vi "Errorbar0007.vi"   [LabVIEW 2013]
uses:
  <vilib>/Heliosphere Research LLC/Advanced Plotting Toolkit/api_plotting/ErrorbarProperties.ctl
  <vilib>/Heliosphere Research LLC/Advanced Plotting Toolkit/typedefs/PlotColor.ctl
  <vilib>/Heliosphere Research LLC/Advanced Plotting Toolkit/properties/Display.ctl
  <vilib>/Heliosphere Research LLC/Advanced Plotting Toolkit/api_core/NewPlotScales.ctl
  <vilib>/Heliosphere Research LLC/Advanced Plotting Toolkit/Advanced Plotting Toolkit.lvlib
types:
  T1 = typedef "Advanced Plotting Toolkit.lvlib/NewPlotScales.ctl" = enum16{"Default", "Linear", "Log", "Symlog"}
  T2 = typedef "Advanced Plotting Toolkit.lvlib/ErrorbarProperties.ctl" = cluster{"Color":T3, "Line Width":dbl, "Cap Size":dbl, "Display":T4}
  T3 = typedef "Advanced Plotting Toolkit.lvlib/PlotColor.ctl" = u32
  T4 = typedef "Advanced Plotting Toolkit.lvlib/Display.ctl" = cluster{"Alpha":dbl, "Z Order":dbl}
  T5 = typedef "Advanced Plotting Toolkit.lvlib/PlotID.ctl" = i32
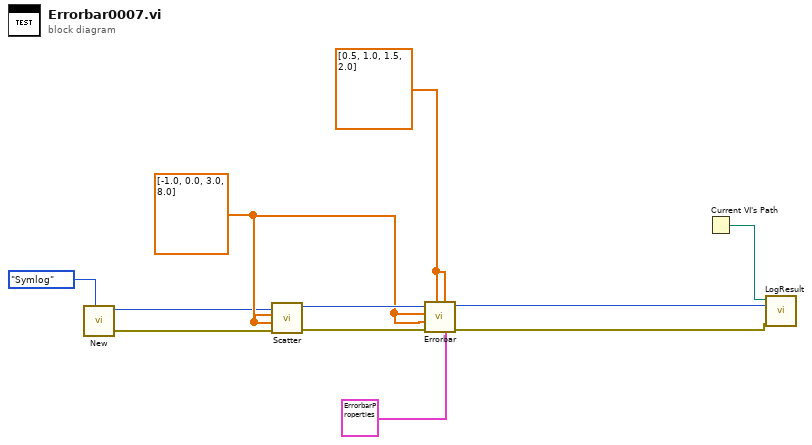
[diagram p0: block diagram]
diagram:
  w5 = dbl[] [0.5, 1.0, 1.5, 2.0] ("X Errors")
  w6 = dbl[] [-1.0, 0.0, 3.0, 8.0] ("X Data")
  n1 = call <vilib>:"New.vi"("X Axis Scale"=NewPlotScales."Symlog") -> ("error out"=w1:errorcluster, "Plot ID"=w2:T5)  [unwired: 9 in]
  n2 = call <vilib>:"Scatter.vi"("error in (no error)"=w1, "Y Data"=w6, "X Data"=w6, "Plot ID"=w2) -> ("error out"=w7:errorcluster, "Plot ID Out"=w8:T5)  [unwired: 6 in]
  n3 = call <vilib>:"Errorbar.vi"("Properties"=T2 {"Color"=2147483647, "Line Width"=nan, "Cap Size"=nan, "Display"={"Alpha"=nan, "Z Order"=nan}} ("Errorbar Properties"), "Y Errors"=w5, "X Errors"=w5, "error in (no error)"=w7, "Y Data"=w6, "X Data"=w6, "Plot ID"=w8) -> ("error out"=w9:errorcluster, "Plot ID out"=w10:T5)  [unwired: 3 in]
  n4 = Current VI's Path() -> (path=w11:path)
  n5 = call "LogResult.vi"("Test Result"=w9, "Test Artifact"=w10, "VI Path"=w11) -> ()  [unwired: 9 in]
